vi "BHBL_integer.vi"(1 "lo(x)":u8 format="%x", 2 "hi(x)":u8 format="%x") -> (0 "(hi.lo)":i16)   [LabVIEW 2011]
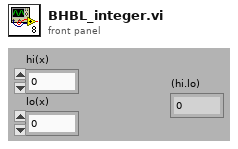
[diagram p1: front panel]
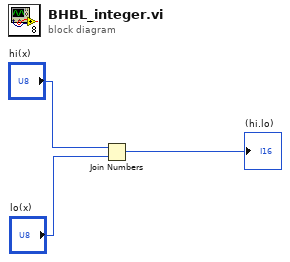
[diagram p0: block diagram]
diagram:
  n1 = Join Numbers(hi="hi(x)", lo="lo(x)") -> ((hi.lo)=→"(hi.lo)":u16)
